vi "AIT 664 - Conditionally Serialize.vi"(8 "error in (no error)":errorcluster, 11 "Device Item Ref in":T1 format="%.0x") -> (0 "error out":errorcluster)   [LabVIEW 2015, in "AIT 664 Custom Device.lvlib"]
uses:
  AIT 664 Custom Device.lvlib
  <vilib>/NI Veristand/Custom Device API/Custom Device Item Ref.ctl
  <vilib>/NI Veristand/Custom Device API/NI VeriStand - Add Custom Device Dependencies.vi
  <vilib>/NI Veristand/Custom Device API/NI VeriStand - Reset Custom Device Dependencies.vi
  <vilib>/NI Veristand/Custom Device API/Get Item Property (Path).vi
  Controls and Global/Global.vi
  <vilib>/NI Veristand/Custom Device API/Custom Device API.lvlib
panel:
  out "Destination File":path
  out "Converted File":path
  out "Value":path
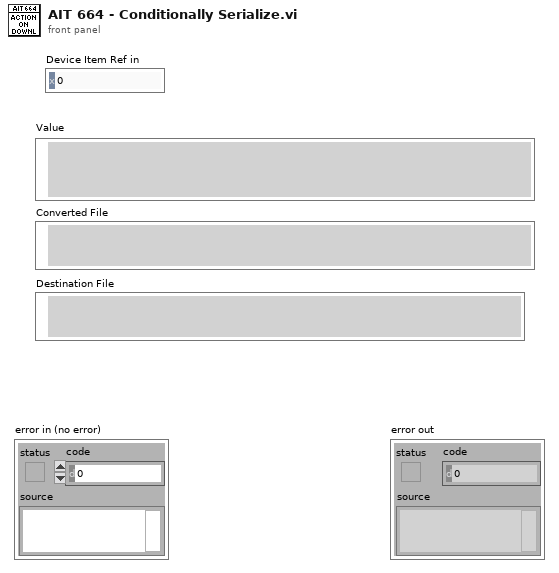
[diagram p1: front panel]
types:
  T1 = typedef "Custom Device API.lvlib/Custom Device Item Ref.ctl" = u64
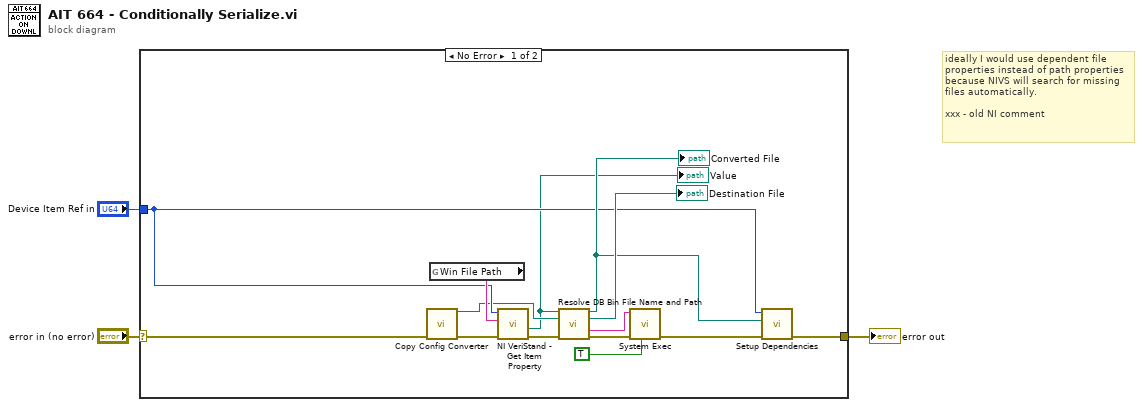
[diagram p0: block diagram]
diagram:
  # "ideally I would use dependent file properties instead of path properties because NIVS will search for missing files automatically.\n\nxxx - old NI comment"
  n1 = case shown="No Error" "error in (no error)" {
    selector: "error in (no error)" -> [w8 w18]
    tunnel: [w5 w18] -> w2
    tunnel: "Device Item Ref in" -> [w9 _]
    frame No Error {
      n2 = call "Copy Config Converter.vi"("error in (no error)"=w8) -> ("path"=w7:path, "error out"=w11:errorcluster)  [unwired: 13 in]
      n3 = global read "Global.vi" "Win File Path"() -> (w17:string)
      n4 = call-poly <vilib>:"NI VeriStand - Get Item Property.vi"("error in (no error)"=w11, "Property Name"=w17, "Item Ref in"=w9) -> ("error out"=w15:errorcluster, "Value"=w6:path)  [unwired: 5 in, 2 out]
      "Value" <- w6
      n5 = call "Resolve DB Bin File Name and Path.vi"("DB XML File"=w6, "Path to Tools"=w7, "error in"=w15) -> ("Converted File"=w10:path, "Destination File"=→"Destination File":path, "SysExec"=w4:string, "error out"=w14:errorcluster)  [unwired: 9 in]
      "Converted File" <- w10
      n6 = call <vilib>:"System Exec.vi"("run minimized? (F)"=TRUE, "error in (no error)"=w14, "command line"=w4) -> ("error out"=w13:errorcluster)  [unwired: 5 in, 3 out]
      n7 = call "Setup Dependencies.vi"("error in (no error)"=w13, "Windows Bin File"=w10, "Item Ref in"=w9) -> ("error out"=w5:errorcluster)  [unwired: 8 in]
    }
    frame Error {
    }
  }
  "error out" <- w2
